vi "Read rotatorFrame.vi"(8 "error in (no error)":errorcluster, 11 "Rotator in":refnum<class "Rotator.lvclass">) -> (0 "error out":errorcluster, 2 "rotatorFrame":T1, 3 "Rotator out":refnum<class "Rotator.lvclass">)   [LabVIEW 2022 SP3, in "TCSDataDefinitions.lvlib" / "TCSCommand.lvlib" / "TargetConfiguration.lvlib" / "Rotator.lvclass"]
uses:
  Rotator.lvclass
  RotatorCommands/Enumerations/RotatorFrameValues.ctl
  Rotator.lvclass/Rotator.ctl
  TCSCommand.lvlib
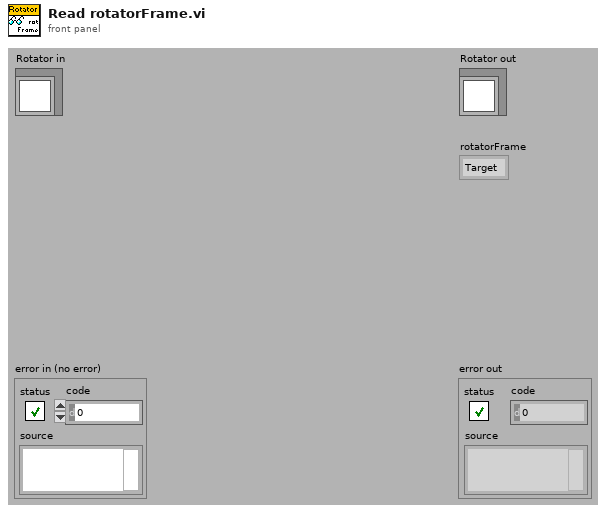
[diagram p1: front panel]
types:
  T1 = typedef "TCSDataDefinitions.lvlib/TCSCommand.lvlib/RotatorFrameValues.ctl" = enum16{"Target", "Fixed"}
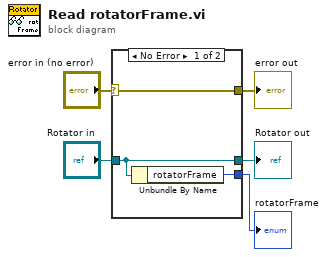
[diagram p0: block diagram]
diagram:
  n1 = case shown="No Error" "error in (no error)" {
    selector: "error in (no error)" -> [w8 w9]
    tunnel: [w8 w9] -> w4
    tunnel: [w7 w10] -> w2
    tunnel: "Rotator in" -> [w7 w10]
    tunnel: [w6 _] -> w1
    frame No Error {
      n2 = Unbundle By Name(w7) -> ("rotatorFrame"=w6:T1)
    }
    frame Error {
    }
  }
  "error out" <- w4
  "Rotator out" <- w2
  "rotatorFrame" <- w1
